vi "Write State.vi"(8 "error in":errorcluster, 10 "State":refnum<class "State Pattern.lvclass">, 11 "Context in":refnum<class "State Pattern.lvclass">) -> (0 "error out":errorcluster, 3 "Context out":refnum<class "State Pattern.lvclass">)   [LabVIEW 2021, in "State Pattern.lvclass"]
uses:
  State Pattern.lvclass
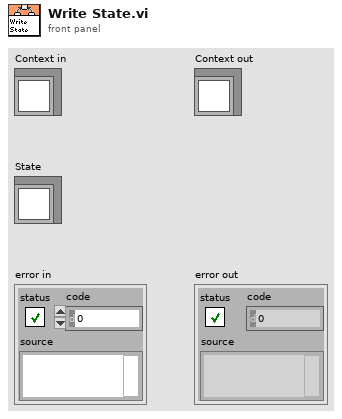
[diagram p1: front panel]
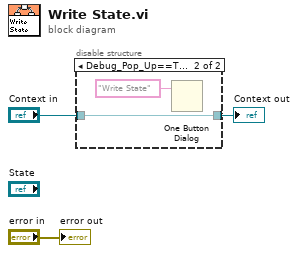
[diagram p0: block diagram]
diagram:
  n1 = disable-structure shown="Debug_Pop_Up==TRUE" {
    disable-tunnel: [w4 w5] -> w1
    disable-tunnel: "Context in" -> [w4 w5]
    frame condition #0 (active) {
    }
    frame condition #1 {
      n2 = One Button Dialog(message="Write State") -> ()  [unwired: 1 in, 1 out]
    }
  }
  "Context out" <- w1
  "error out" <- "error in"
